vi "Compute Calibration Phasor & jw.vi"(4 "Laser Period":dbl[unit], 6 "Gate Width":dbl[unit], 7 "Harmonic frequency":dbl[unit], 8 "Error In":errorcluster, 9 "# Gates":dbl, 10 "Calibration Lifetime":dbl[unit], 11 "Calibration Phasor Type":T1) -> (0 "Error Out":errorcluster, 1 "z (tau_cal)":cdb, 3 "i 2 pi f (GHz)":cdb)   [LabVIEW 2019]
doc: "z (tau_cal) is the phasor calculated for tau_cal in either the UC_00 case (standard universal semicircle) or the UC_N case (discrete phasor of ungated periodic single-exponential decay), depending on the selected Calibration Phasor Type"
uses:
  SEPL Type.ctl
  <vilib>/Utility/error.llb/Error Cluster From Error Code.vi
  <vilib>/ErrorRing/Error Ring.xnode
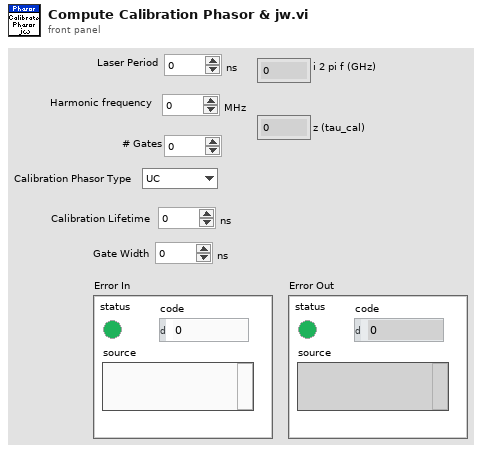
[diagram p1: front panel]
types:
  T1 = typedef "SEPL Type.ctl" = enum16{"UC", "L_N", "L_N[W]", "L_X"}
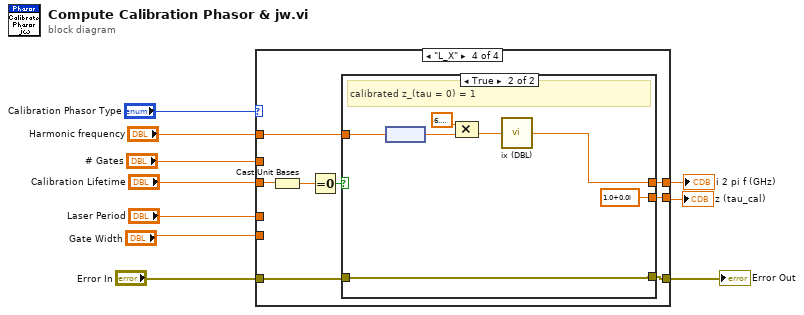
[diagram p0: block diagram]
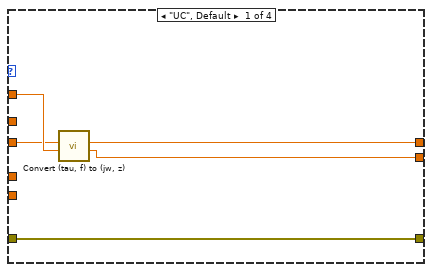
[diagram p2: hidden frame]
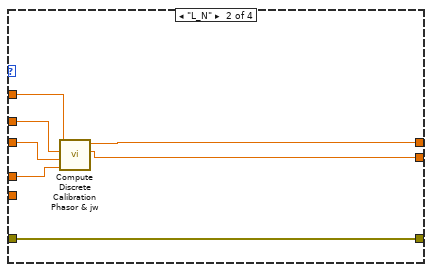
[diagram p3: hidden frame]
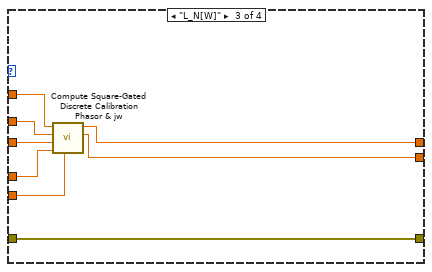
[diagram p4: hidden frame]
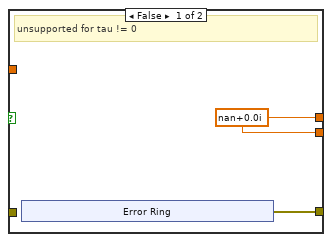
[diagram p5: hidden frame]
diagram:
  n1 = case shown="\"L_X\"" "Calibration Phasor Type" {
    tunnel: "Harmonic frequency" -> [w15 w22 w30 w31]
    tunnel: [w14 w16 w26 w33] -> w5
    tunnel: [w13 w18 w25 w32] -> w6
    tunnel: "Calibration Lifetime" -> [w12 w20 w28 w38]
    tunnel: "# Gates" -> [_ w21 w29 _]
    tunnel: "Laser Period" -> [_ w19 w27 _]
    tunnel: "Gate Width" -> [_ _ w24 _]
    tunnel: "Error In" -> [w11 w17 w23 w35]
    tunnel: [w11 w17 w23 w34] -> w1
    frame "UC", Default {
      n2 = call "Convert (tau, f) to (jw, z).vi"("Harmonic Frequency"=w15, "Lifetime"=w12) -> ("Phasor"=w13:cdb, "i 2 pi f (GHz)"=w14:cdb)  [unwired: 8 in]
    }
    frame "L_N" {
      n3 = call "Compute Discrete Calibration Phasor & jw.vi"("Laser Period (T)"=w19, "Calibration Lifetime (tau)"=w20, "# Gates (N)"=w21, "Harmonic frequency (f)"=w22) -> ("Z_N(tau)"=w18:cdb, "i 2 pi f (GHz)"=w16:cdb)  [unwired: 6 in]
    }
    frame "L_N[W]" {
      n4 = call "Compute Square-Gated Discrete Calibration Phasor & jw.vi"("Gate Width (W)"=w24, "Laser Period (T)"=w27, "Calibration Lifetime (tau)"=w28, "# Gates (N)"=w29, "Harmonic frequency (f)"=w30) -> ("Z_N[W](tau)"=w25:cdb, "i 2 pi f (GHz)"=w26:cdb)  [unwired: 5 in]
    }
    frame "L_X" {
      n5 = Cast Unit Bases(0:w38) -> (2:w37:dbl)  [unwired: 1 in]
      n6 = Equal To 0?(x=w37) -> (x = 0?=w36:bool)
      n7 = case shown="True" w36 {
        tunnel: w35 -> [_ w51]
        tunnel: [w40 w51] -> w34
        tunnel: [w39 w46] -> w33
        tunnel: [w39 cdb 1.0+0.0i ("i 2 pi f (GHz)")] -> w32
        tunnel: w31 -> [_ w47]
        frame False {
          w39 = cdb nan+0.0i ("i 2 pi f (GHz)")
          # "unsupported for tau != 0"
          n8 = xnode "Error Ring"() -> ("error out"=w40:errorcluster)
        }
        frame True {
          # "calibrated z_(tau = 0) = 1"
          n9 = node(w47) -> (w49:dbl)
          n10 = Compound Arithmetic op=MULTIPLY(6.283185307179586, w49) -> (w48:dbl)
          n11 = call "ix (DBL).vi"("x (1)"=w48) -> ("i.(x)"=w46:cdb)
        }
      }
    }
  }
  "z (tau_cal)" <- w6
  "i 2 pi f (GHz)" <- w5
  "Error Out" <- w1
